vi "GetTrendPointProps.vi"(7 "data event":T1, 9 "hw status":string, 10 "found hw status":bool, 11 "DataSetName":string) -> (3 "key value pairs out":T7[](array[typedef]))   [LabVIEW 2017, in "DataEventCreator.lvlib"]
uses:
  <vilib>/addons/InsightCM/Devices/Shared/Common/DataEventCreator/DataEventCreator.lvlib
  <vilib>/addons/InsightCM/MessageBus/Base/controls/KeyValuePair.ctl
  <vilib>/addons/InsightCM/Devices/Shared/Cms/CmsDataEventCreator/controls/DataEventConfig.ctl
  <vilib>/addons/InsightCM/Devices/Shared/Cms/CmsDataEventCreator/controls/AcqParams.ctl
  <vilib>/addons/InsightCM/Devices/Shared/Common/DataAccumulator/controls/AccumulationSettings.ctl
  <vilib>/addons/InsightCM/Devices/Shared/Common/DataAccumulator/controls/accumulationType.ctl
  <vilib>/addons/InsightCM/Devices/Shared/Common/DVRBuffer/controls/BufferLocation.ctl
  <vilib>/addons/PointValueMap/controls/PointMap.ctl
  <vilib>/addons/InsightCM/Devices/Shared/Common/DataEvent/controls/DataSetType.ctl
  <vilib>/addons/InsightCM/Utilities/PropertyHelpers/PropertyHelpers.lvlib
  <vilib>/addons/InsightCM/Devices/Shared/Common/DataEvent/DataEvent.lvlib
  <vilib>/addons/InsightCM/Devices/Shared/Common/DataAccumulator/DataAccumulator.lvlib
  <vilib>/addons/InsightCM/Devices/Shared/Common/DVRBuffer/DVRBuffer.lvlib
  <vilib>/addons/InsightCM/Devices/Shared/Cms/CmsDataEventCreator/CmsDataEventCreator.lvlib
  <vilib>/addons/PointValueMap/PointValueMap.lvlib
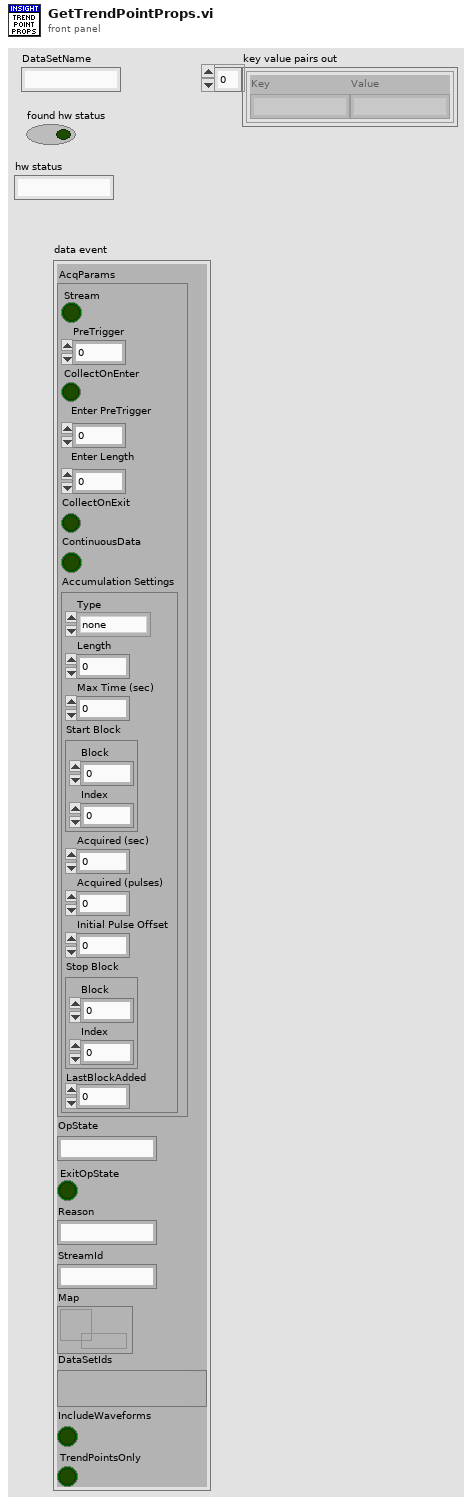
[diagram p1: front panel]
types:
  T1 = typedef "CmsDataEventCreator.lvlib/DataEventConfig.ctl" = cluster{"AcqParams":T2, "OpState":string, "ExitOpState":bool, "Reason":string, "StreamId":string, "Map":T6, "DataSetIds":variant, "IncludeWaveforms":bool, "TrendPointsOnly":bool}
  T2 = typedef "CmsDataEventCreator.lvlib/AcqParams.ctl" = cluster{"Stream":bool, "PreTrigger":i32, "CollectOnEnter":bool, "Enter PreTrigger":i32, "Enter Length":dbl, "CollectOnExit":bool, "ContinuousData":bool, "Accumulation Settings":T3}
  T3 = typedef "DataAccumulator.lvlib/AccumulationSettings.ctl" = cluster{"Type":T4, "Length":dbl, "Max Time (sec)":dbl, "Start Block":T5, "Acquired (sec)":dbl, "Acquired (pulses)":i32, "Initial Pulse Offset":dbl, "Stop Block":T5, "LastBlockAdded":u32}
  T4 = typedef "DataAccumulator.lvlib/accumulationType.ctl" = enum16{"none", "seconds", "revolutions"}
  T5 = typedef "DVRBuffer.lvlib/BufferLocation.ctl" = cluster{"Block":u32, "Index":i32}
  T6 = typedef "PointValueMap.lvlib/PointMap.ctl" = refnum<data-value>
  T7 = typedef "KeyValuePair.ctl" = cluster{"Key":string, "Value":string}
  T8 = typedef "DataEvent.lvlib/DataSetType.ctl" = enum16{"Waveform", "SpeedProfile", "ThermalImage", "EmsaSweep"}
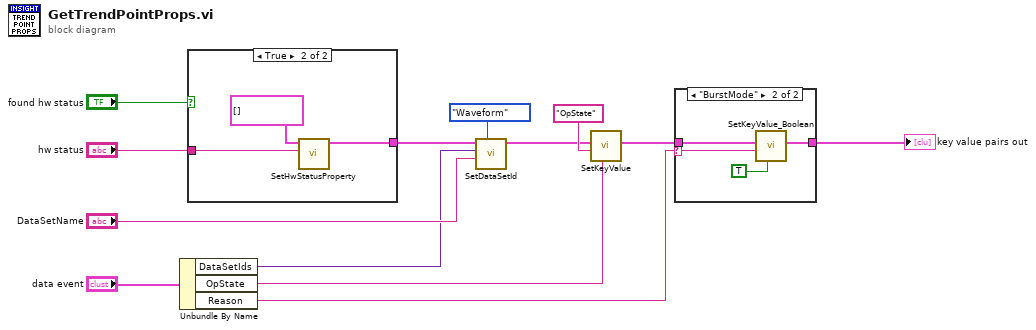
[diagram p0: block diagram]
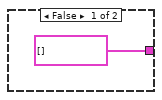
[diagram p3: hidden frame]
diagram:
  n1 = Unbundle By Name("data event") -> ("DataSetIds"=w7:variant, "OpState"=w6:string, "Reason"=w1:string)
  n2 = case shown="True" "found hw status" {
    tunnel: [T7[] [] ("props out") w17] -> w12
    tunnel: "hw status" -> [_ w16]
    frame False {
    }
    frame True {
      n3 = call <vilib>:"SetHwStatusProperty.vi"("hw status"=w16, "props in"=T7[] []) -> ("props out"=w17:T7[])  [unwired: 9 in]
    }
  }
  n4 = call <vilib>:"SetDataSetId.vi"("DataSetType"=DataSetType."Waveform", "DataSetName"="DataSetName", "DataSetIds"=w7, "props in"=w12) -> ("props out"=w10:T7[])  [unwired: 7 in]
  n5 = call <vilib>:"SetKeyValue.vi"("value"=w6, "key"="OpState", "key value pairs"=w10) -> ("key value pairs out"=w3:T7[])  [unwired: 8 in]
  n6 = case shown="\"BurstMode\"" w1 {
    selector: w1 -> [_ w20]
    tunnel: w3 -> [w18 w22]
    tunnel: [w18 w21] -> w2
    frame Default {
    }
    frame "BurstMode" {
      n7 = call <vilib>:"SetKeyValue_Boolean.vi"("value"=TRUE, "key"=w20, "key value pairs"=w22) -> ("key value pairs out"=w21:T7[])  [unwired: 8 in]
    }
  }
  "key value pairs out" <- w2
